vi "setIRQ.vi"(10 "IRQ":refnum<class "IIRQ.lvclass">, 11 "Modbus in":refnum<class "Modbus.lvclass">) -> (3 "Modbus out":refnum<class "Modbus.lvclass">)   [LabVIEW 2016, in "RTModbusFPGA.lvlib" / "Modbus.lvclass"]
uses:
  Modbus.lvclass
  Common_RT_FPGA/IIRQ/IIRQ.lvclass
  Modbus.lvclass/Modbus.ctl
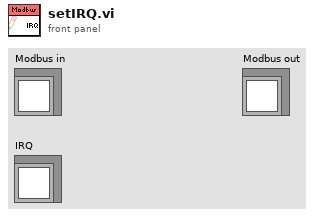
[diagram p1: front panel]
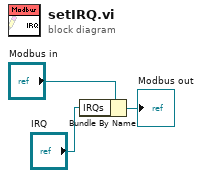
[diagram p0: block diagram]
diagram:
  n1 = Bundle By Name(cluster="Modbus in", "IRQs"="IRQ") -> (→"Modbus out":refnum<class "Modbus.lvclass">)
